vi "Gas Correction Factor.vi"(7 "Set? (F:Read)":bool, 8 "Error In":errorcluster, 9 "Gas Correction Factor (100%)":dbl=100.0, 10 "Channel (0)":i32, 11 "VISA resource name":refnum<visa-resource-name>) -> (0 "Error Out":errorcluster, 1 "Gas Correction Factor out":dbl, 3 "dup VISA resource name":refnum<visa-resource-name>)   [LabVIEW 2011, in "MGC647C.lvlib"]
doc: "Read/Set gas correction factor."
uses:
  <instrlib>/MGC647C/MGC647C.lvlib
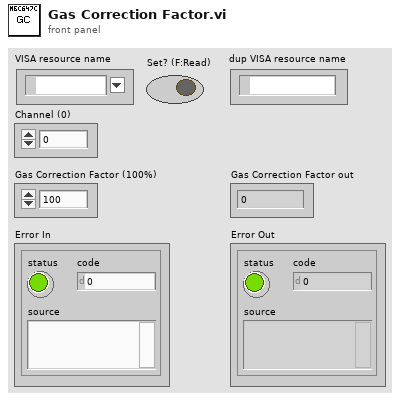
[diagram p1: front panel]
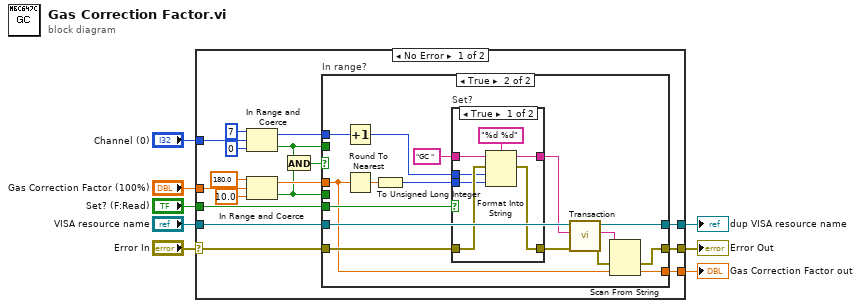
[diagram p0: block diagram]
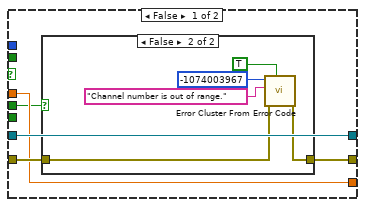
[diagram p2: hidden frame]
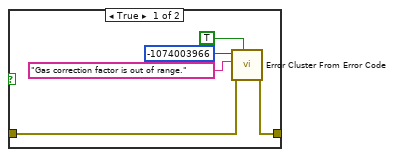
[diagram p3: hidden frame]
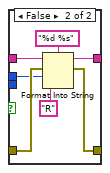
[diagram p4: hidden frame]
diagram:
  n1 = case shown="No Error" "Error In" {
    selector: "Error In" -> [w17 w72]
    tunnel: "VISA resource name" -> [w25 w71]
    tunnel: [w24 w71] -> w7
    tunnel: [w23 w72] -> w6
    tunnel: "Set? (F:Read)" -> [w22 _]
    tunnel: "Gas Correction Factor (100%)" -> [w21 w73]
    tunnel: [w16 w73] -> w2
    tunnel: "Channel (0)" -> [w13 _]
    frame No Error {
      n2 = In Range and Coerce(upper limit=7, x=w13, lower limit=0) -> (coerced(x)=w12:i32, In Range?=w10:bool)
      n3 = In Range and Coerce(upper limit=180.0, x=w21, lower limit=10.0) -> (coerced(x)=w20:dbl, In Range?=w9:bool)
      n4 = And(x=w10, y=w9) -> (x .and. y?=w11:bool)
      n5 = case "In range?" shown="True" w11 {
        tunnel: w25 -> [w28 w56]
        tunnel: [w28 w55] -> w24
        tunnel: [w29 w50] -> w23
        tunnel: w22 -> [_ w43]
        tunnel: w20 -> [w27 w42]
        tunnel: w17 -> [w30 w54]
        tunnel: [w27 w41] -> w16
        tunnel: w12 -> [_ w49]
        tunnel: w10 -> [_ _]
        tunnel: w9 -> [w26 _]
        frame False {
          n6 = case shown="False" w26 {
            tunnel: w30 -> [w35 w40]
            tunnel: [w34 w39] -> w29
            frame True {
              n7 = call <vilib>:"Error Cluster From Error Code.vi"("show call chain? (False)"=TRUE, "error in (no error)"=w35, "error message (\"\")"="Gas correction factor is out of range." ("error message (\"\")"), "error code (0)"=-1074003966) -> ("error out"=w34:errorcluster)  [unwired: 5 in]
            }
            frame False {
              n8 = call <vilib>:"Error Cluster From Error Code.vi"("show call chain? (False)"=TRUE, "error in (no error)"=w40, "error message (\"\")"="Channel number is out of range." ("error message (\"\")"), "error code (0)"=-1074003967) -> ("error out"=w39:errorcluster)  [unwired: 5 in]
            }
          }
        }
        frame True {
          n9 = Increment(x=w49) -> (x+1=w48:i32)
          n10 = Round To Nearest(number=w42) -> (nearest integer value=w47:dbl)
          n11 = To Unsigned Long Integer(number=w47) -> (unsigned 32bit integer=w46:u32)
          n12 = case "Set?" shown="True" w43 {
            tunnel: w54 -> [w63 w70]
            tunnel: [w62 w69] -> w53
            tunnel: w48 -> [w61 w68]
            tunnel: w46 -> [w60 _]
            tunnel: "GC " ("string (\"\")") -> [w59 w67]
            tunnel: [w58 w66] -> w44
            frame True {
              n13 = Format Into String(format string="%d %d", initial string=w59, error in=w63, w61, w60) -> (resulting string=w58:string, error out=w62:errorcluster)
            }
            frame False {
              n14 = Format Into String(format string="%d %s", initial string=w67, error in=w70, w68, "R") -> (resulting string=w66:string, error out=w69:errorcluster)
            }
          }
          n15 = call <instrlib>:"Transaction.vi"("Error In"=w53, "Command"=w44, "VISA resource name"=w56) -> ("Error Out"=w51:errorcluster, "Response"=w52:string, "dup VISA resource name"=w55:refnum<visa-resource-name>)  [unwired: 6 in]
          n16 = Scan From String(input string=w52, error in=w51, default 1=w42) -> (error out=w50:errorcluster, output 1=w41:dbl)  [unwired: 2 in, 2 out]
        }
      }
    }
    frame Error {
    }
  }
  "dup VISA resource name" <- w7
  "Error Out" <- w6
  "Gas Correction Factor out" <- w2
